vi "Read Id_b.vi"(10 "write string":string="id\r" caption="wlaczona opcja \"codes display\"", 11 "VISA resource name":refnum<visa-resource-name>="COM7") -> (2 "read string":string)   [LabVIEW 2017]
panel:
  # "wlaczona opcja \"codes display\""
  # "wlaczona opcja \"codes display\""
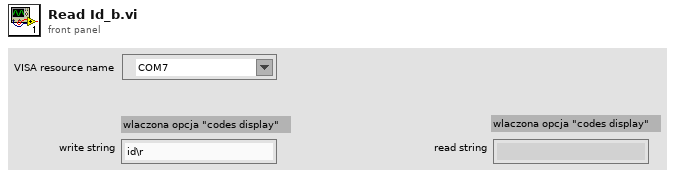
[diagram p1: front panel]
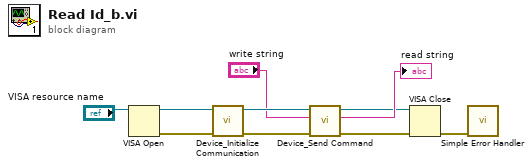
[diagram p0: block diagram]
diagram:
  n1 = VISA Open(VISA resource name="VISA resource name") -> (VISA resource name=w9:refnum<visa-resource-name>, error out=w8:errorcluster)  [unwired: 4 in]
  n2 = call "Device_Initialize Communication.vi"("error in (no error)"=w8, "VISA Refnum in"=w9) -> ("error out"=w7:errorcluster, "VISA Refnum out"=w6:refnum<visa-resource-name>)  [unwired: 8 in]
  n3 = call "Device_Send Command.vi"("error in (no error)"=w7, "write string"="write string", "VISA Refnum in"=w6) -> ("error out"=w3:errorcluster, "read buffer"=→"read string":string, "VISA Refnum out"=w2:refnum<visa-resource-name>)  [unwired: 6 in]
  n4 = VISA Close(VISA resource name=w2, error in (no error)=w3) -> (error out=w1:errorcluster)
  n5 = call <vilib>:"Simple Error Handler.vi"("error in (no error)"=w1) -> ()  [unwired: 4 in, 5 out]
